vi "Connections to Strings.vi"(8 "error in":errorcluster, 10 "connection list":T2[](array[typedef]), 11 "routing and faulting in":T1 format="%.0x") -> (0 "error out":errorcluster, 2 "connection strings":string[](array[string]), 3 "routing and faulting out":T1 format="%.0x")   [LabVIEW 2020, in "Routing and Faulting Scripting.lvlib"]
uses:
  Routing and Faulting Scripting.lvlib
  Shared/Connection.ctl
  <vilib>/NI VeriStand/Custom Device API/Custom Device Item Ref.ctl
  Shared/Routing and Faulting Shared.lvlib
  <vilib>/NI VeriStand/Custom Device API/Custom Device API.lvlib
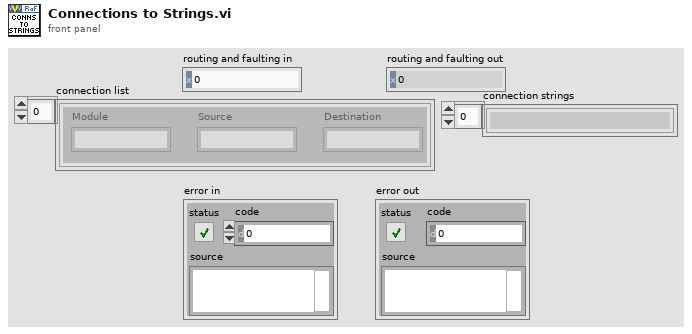
[diagram p1: front panel]
types:
  T1 = typedef "Custom Device API.lvlib/Custom Device Item Ref.ctl" = u64
  T2 = typedef "Routing and Faulting Shared.lvlib/Connection.ctl" = cluster{"Module":string, "Source":string, "Destination":string}
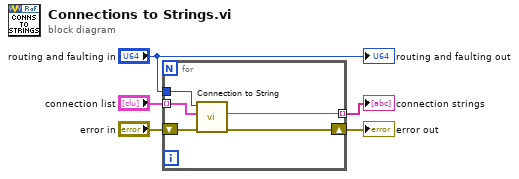
[diagram p0: block diagram]
diagram:
  n1 = for {
    tunnel: "connection list" -> [w10] mode=indexing
    tunnel: [w9] -> w4 mode=indexing
    shift-right: [w7] -> w2
    shift-left: "error in" -> [w8]
    tunnel: "routing and faulting in" -> [w6]
    n2 = call "Connection to String.vi"("error in"=w8, "connection"=w10, "routing and faulting in"=w6) -> ("error out"=w7:errorcluster, "string"=w9:string)  [unwired: 5 in, 2 out]
  }
  "connection strings" <- w4
  "error out" <- w2
  "routing and faulting out" <- "routing and faulting in"
